vi "Pre Launch Init.vi"(11 "Nested in":refnum<class "Stage Controller.lvclass">) -> (0 "error out":errorcluster, 3 "Nested out":refnum<class "Stage Controller.lvclass">)   [LabVIEW 2020, in "Stage.lvlib" / "Stage Controller.lvlib" / "Stage Controller.lvclass"]
doc: "(<B>Filename</B>: Actor Framework.lvlib:Actor.lvclass:Pre Launch Init.vi)\n\nDefines behavior that occurs after the Launch Nested Actor method is invoked but before the actor's Actor Core method begins running.\n\nBy default, this method does nothing. A descendant class may override it to define behavior."
uses:
  Stage Controller.lvclass
  Stage Controller.lvclass/Stage Controller.ctl
  <vilib>/ActorFramework/Actor/Actor.lvclass
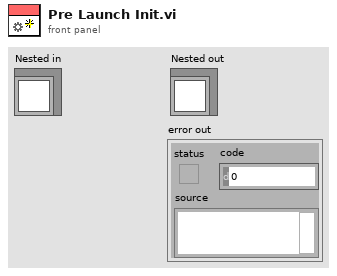
[diagram p1: front panel]
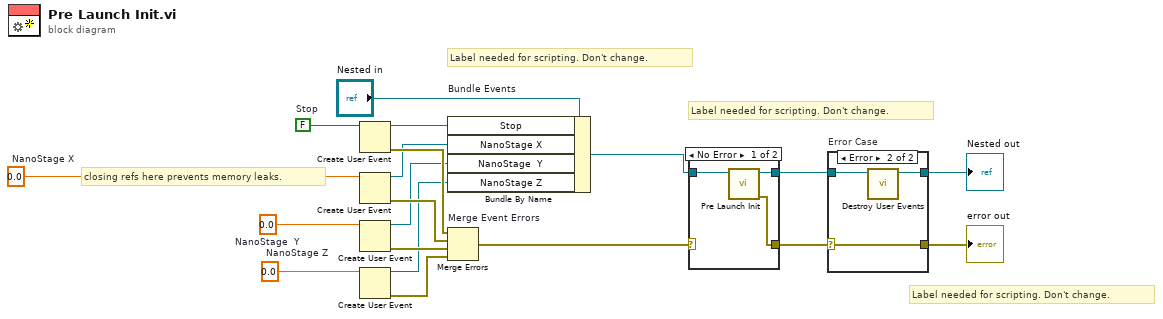
[diagram p0: block diagram]
diagram:
  w3 = 0.0  # NanoStage Z
  w6 = 0.0  # NanoStage  Y
  w9 = 0.0  # NanoStage X
  w18 = FALSE  # Stop
  # "Label needed for scripting. Don't change."
  # "Label needed for scripting. Don't change."
  # "Label needed for scripting. Don't change."
  # "closing refs here prevents memory leaks."
  n1 = Create User Event(user event datatype=w18) -> (user event=w15:refnum<user-event>, error out=w17:errorcluster)  [unwired: 1 in]
  n2 = Create User Event(user event datatype=w9) -> (user event=w8:refnum<user-event>, error out=w7:errorcluster)  [unwired: 1 in]
  n3 = Create User Event(user event datatype=w6) -> (user event=w5:refnum<user-event>, error out=w4:errorcluster)  [unwired: 1 in]
  n4 = Create User Event(user event datatype=w3) -> (user event=w2:refnum<user-event>, error out=w1:errorcluster)  [unwired: 1 in]
  n5 = Bundle By Name "Bundle Events"(cluster="Nested in", "Stop"=w15, "NanoStage X"=w8, "NanoStage  Y"=w5, "NanoStage Z"=w2) -> (w12:refnum<class "Stage Controller.lvclass">)
  n6 = Merge Errors "Merge Event Errors"(w17, w7, w4, w1) -> (w11:errorcluster)
  n7 = case shown="No Error" w11 {
    selector: w11 -> [_ w24]
    tunnel: [w22 w23] -> w13
    tunnel: w12 -> [w21 w23]
    tunnel: [w20 w24] -> w10
    frame No Error {
      n8 = call-parent "Pre Launch Init.vi"("Actor in"=w21) -> ("error out"=w20:errorcluster, "Actor out"=w22:refnum<class "Stage Controller.lvclass">)  [unwired: 9 in]
    }
    frame Error {
    }
  }
  n9 = case "Error Case" shown="Error" w10 {
    selector: w10 -> [w25 w29]
    tunnel: w13 -> [w26 w28]
    tunnel: [w26 w27] -> w16
    tunnel: [w25 w29] -> w14
    frame No Error {
    }
    frame Error {
      n10 = call "Destroy User Events.vi"("UI Template in"=w28) -> ("UI Template out"=w27:refnum<class "Stage Controller.lvclass">)  [unwired: 10 in]
    }
  }
  "error out" <- w14
  "Nested out" <- w16
